vi "Reverse number_0.vi"() -> ()   [LabVIEW 2015]
panel:
  in  "Tab Control":enum32{"Page 1", "Page 2"}(tab)
  in  "help of User Value":i64
  out "Reverse value":i64
  # "Reverse Number"
  # "Pardeep Kumar"
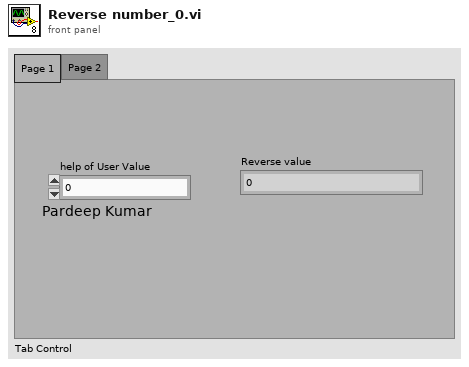
[diagram p1: front panel]
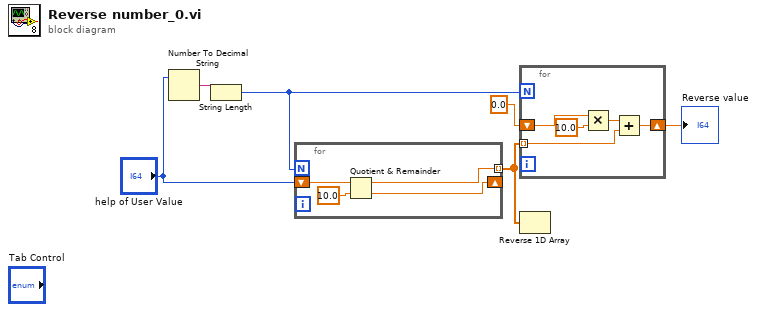
[diagram p0: block diagram]
diagram:
  n1 = Number To Decimal String(number="help of User Value") -> (decimal integer string=w6:string)  [unwired: 1 in]
  n2 = String Length(string=w6) -> (length=w4:i32)
  n3 = for {
    N: w4 -> [_]
    tunnel: [w9] -> w3 mode=indexing
    shift-right: [w8] -> _
    shift-left: "help of User Value" -> [w10]
    n4 = Quotient & Remainder(x=w10, y=10.0) -> (x-y*floor(x/y)=w9:dbl, floor(x/y)=w8:dbl)
  }
  n5 = for {
    N: w4 -> [_]
    tunnel: w3 -> [w13] mode=indexing
    shift-right: [w12] -> w1
    shift-left: 0.0 -> [w11]
    n6 = Multiply(x=w11, y=10.0) -> (x*y=w15:dbl)
    n7 = Add(x=w15, y=w13) -> (x+y=w12:dbl)
  }
  "Reverse value" <- w1
  n8 = Reverse 1D Array(array=w3) -> ()  [unwired: 1 out]
